vi "Error.Clear.vi"(5 "Top of Q":bool, 7 "Q Name":string, 8 "Error In":errorcluster, 11 "Q In":refnum<queue>) -> (0 "Error Out":errorcluster, 3 "Q Out":refnum<queue>)   [LabVIEW 2024, in "EQMF.lvlib" / "Errors.lvlib"]
uses:
  <vilib>/KATE/Queues/Q.Element.ctl
  Errors.lvlib
  <vilib>/KATE/Queues/Queue Utils.lvlib
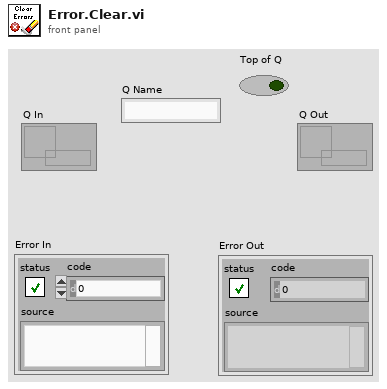
[diagram p1: front panel]
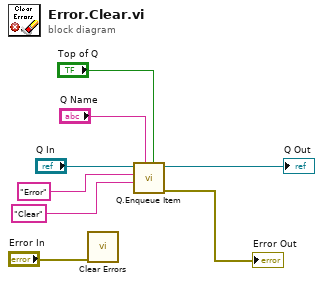
[diagram p0: block diagram]
diagram:
  n1 = call <vilib>:"Clear Errors.vi"("error in (no error)"="Error In") -> ()  [unwired: 5 in, 2 out]
  n2 = call <vilib>:"Q.Enqueue Item.vi"("Top of Q"="Top of Q", "Q Name"="Q Name", "Sub"="Clear" ("Cmd"), "Cmd"="Error", "Q In"="Q In") -> ("error out"=→"Error Out":errorcluster, "Q Out"=→"Q Out":refnum<queue>)  [unwired: 5 in]
